vi "_TangoSubscribeAttributeDataReadyEvent.vi"(1 "error in":errorcluster, 2 "attribute name":string, 3 "device name":string, 4 "attribute data ready event ref":T1) -> (0 "error out":errorcluster)   [LabVIEW 2014, in "tango.lvlib"]
uses:
  tango.lvlib
  Common VIs/Typedefs/_AttributeDataReadyEventRef.ctl
  tango_binding.so
panel:
  out "evt identifier":i32
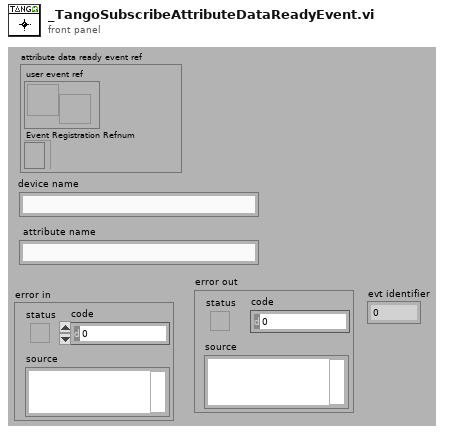
[diagram p1: front panel]
types:
  T1 = typedef "tango.lvlib/_AttributeDataReadyEventRef.ctl" = cluster{"user event ref":refnum<user-event>, "user event reg refnum":refnum<event-registration>}
  T2 = enum32{"CHANGE_EVENT", "DEPRECATED_QUALITY_EVENT", "PERIODIC_EVENT", "ARCHIVE_EVENT", "USER_EVENT", "ATTRIBUTE_CONF_EVENT", "DATA_READY_EVENT", "INTERFACE_CHANGE_EVENT", "UNKNOWN_EVENT"}
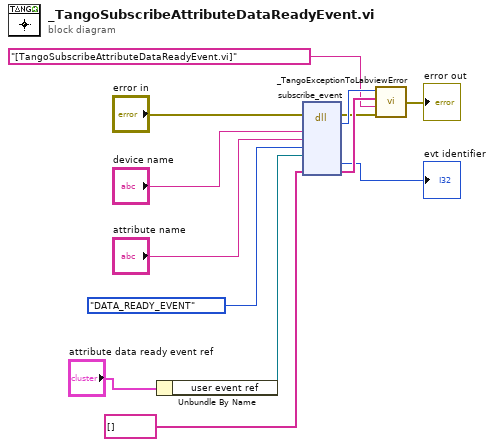
[diagram p0: block diagram]
diagram:
  n1 = Unbundle By Name("attribute data ready event ref") -> ("user event ref"=w4:refnum<user-event>)
  n2 = dll-call lib="tango_binding.*" fn="subscribe_event"(error in="error in", "dev_name"="device name", "attr_name"="attribute name", "evt_type"=T2."DATA_READY_EVENT", "evt_ref"=w4, "error_stack_"=string[] [] ("subscribe error stack")) -> (error out=w7:errorcluster, "return type"=w10:i32, "evt_identifier"=→"evt identifier":i32, "error_stack_"=w9:string[])  [unwired: 7 in, 1 out]
  n3 = call "_TangoExceptionToLabviewError.vi"("error in"=w7, "location"="[TangoSubscribeAttributeDataReadyEvent.vi]", "error stack"=w9, "error code"=w10) -> ("error out"=→"error out":errorcluster)
